vi "AsciiToInt.vi"(9 "offset":i32, 11 "string byte array":u8[](array[numeric])) -> (1 "new offset":i32, 3 "value":i32)   [LabVIEW 2018]
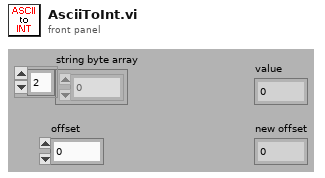
[diagram p1: front panel]
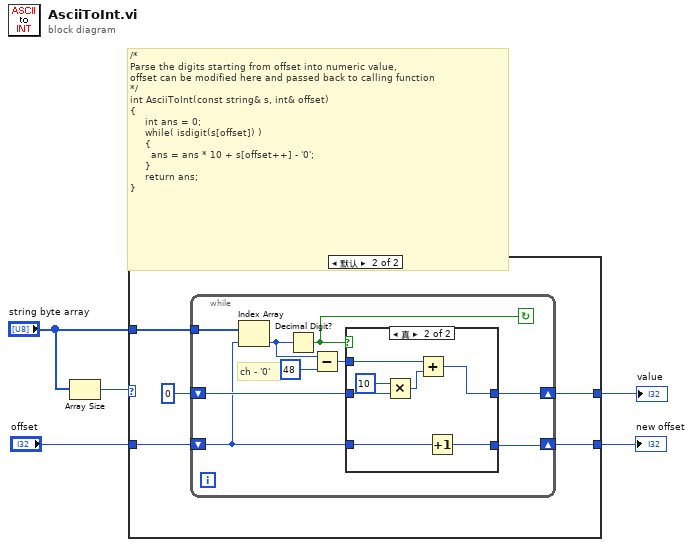
[diagram p0: block diagram]
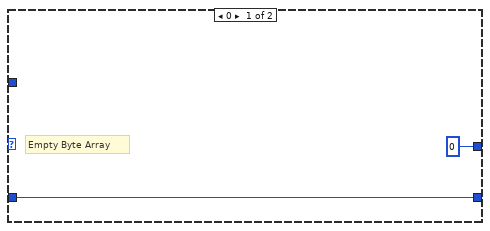
[diagram p2: hidden frame]
diagram:
  # "/* \nParse the digits starting from offset into numeric value,\noffset can be modified here and passed back to calling function \n*/\nint AsciiToInt(const string& s, int& offset)\n{\n    \tint ans = 0;\n\t    while( isdigit(s[offset]) )\n    \t{\n     \t\tans = ans * 10 + s[offset++] - '0';\n    \t}\n    \treturn ans;\n}"
  n1 = Array Size(array="string byte array") -> (size(s)=w5:i32)
  n2 = case shown="默认" w5 {
    tunnel: [w7 w9] -> w4
    tunnel: "offset" -> [w7 w11]
    tunnel: [0 ("value") w8] -> w2
    tunnel: "string byte array" -> [_ w12]
    frame 0 {
      # "Empty Byte Array"
    }
    frame Default {
      n3 = while {
        tunnel: w12 -> [w21]
        shift-right: [w14] -> w9
        shift-left: w11 -> [w13]
        shift-right: [w18] -> w8
        shift-left: 0 -> [w19]
        stop <- w20 continue-if-true
        # "ch - '0'"
        n4 = Index Array(array=w21, index=w13) -> (element=w16:u8)
        n5 = Decimal Digit?(1:w16) -> (0:w20:bool)
        n6 = Subtract(x=w16, y=u8 48) -> (x-y=w17:u8)
        n7 = case shown="真" w20 {
          tunnel: w17 -> [_ w30]
          tunnel: w19 -> [w23 w28]
          tunnel: [w23 w26] -> w18
          tunnel: [w22 w25] -> w14
          tunnel: w13 -> [w22 w24]
          frame False {
            # "if not digit, keep \nprev numeric value"
          }
          frame True {
            n8 = Multiply(x=10, y=w28) -> (x*y=w29:i32)
            n9 = Add(x=w30, y=w29) -> (x+y=w26:i32)
            n10 = Increment(x=w24) -> (x+1=w25:i32)
          }
        }
      }
    }
  }
  "new offset" <- w4
  "value" <- w2
